vi "UNITEST MAIN v2.0.vi"() -> ()   [LabVIEW 2025] (continued)
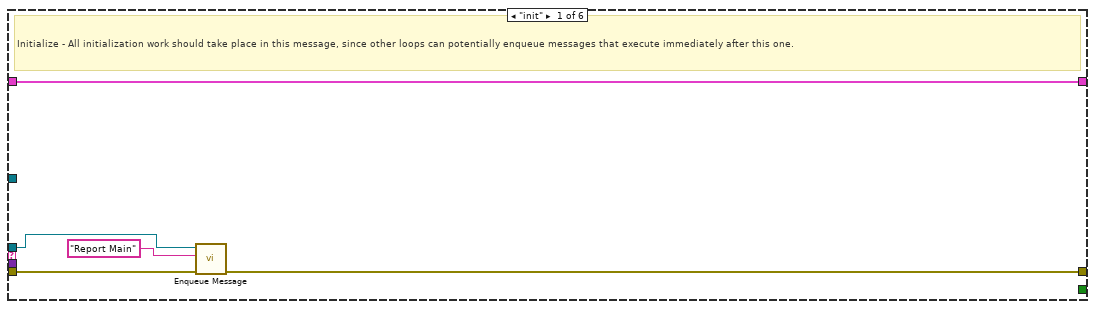
[diagram p2: hidden frame]
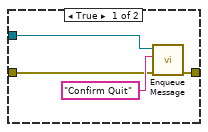
[diagram p3: hidden frame]
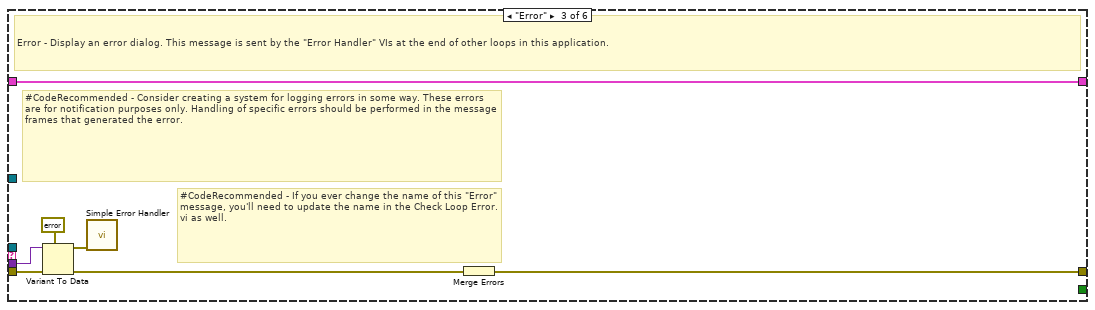
[diagram p4: hidden frame]
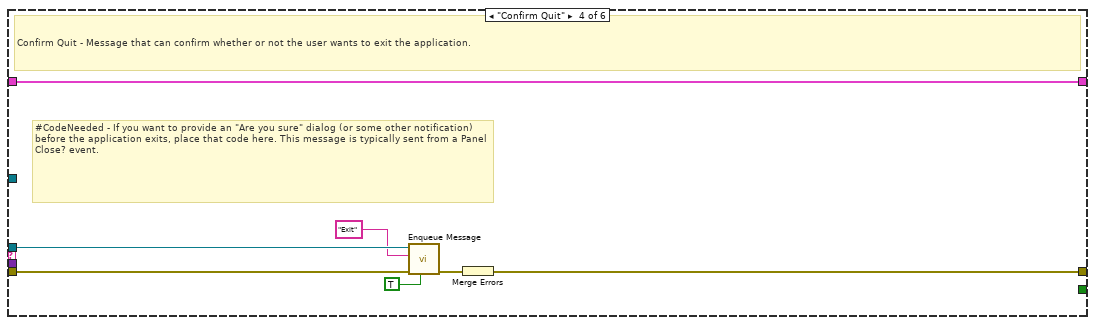
[diagram p5: hidden frame]
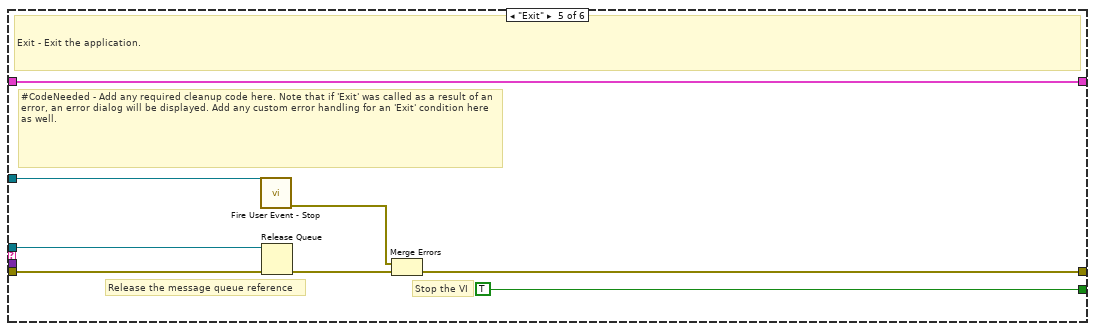
[diagram p6: hidden frame]
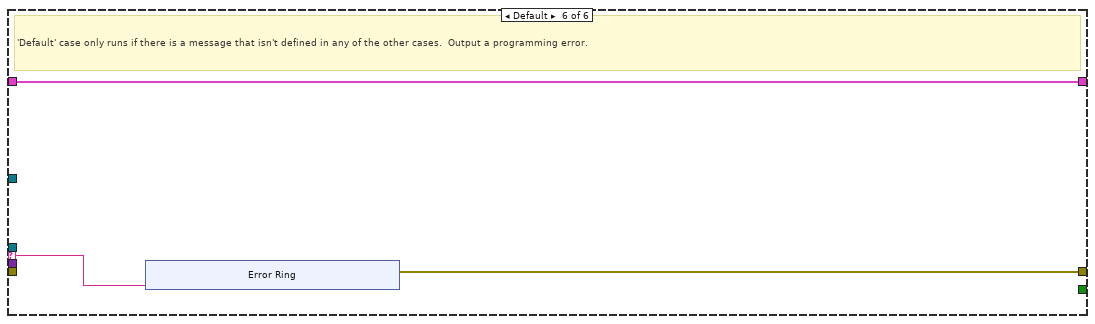
[diagram p7: hidden frame]
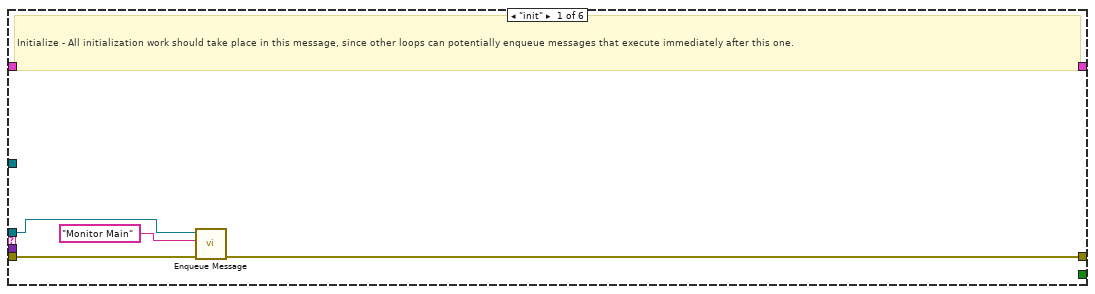
[diagram p8: hidden frame]
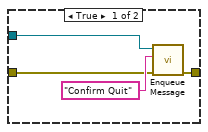
[diagram p9: hidden frame]
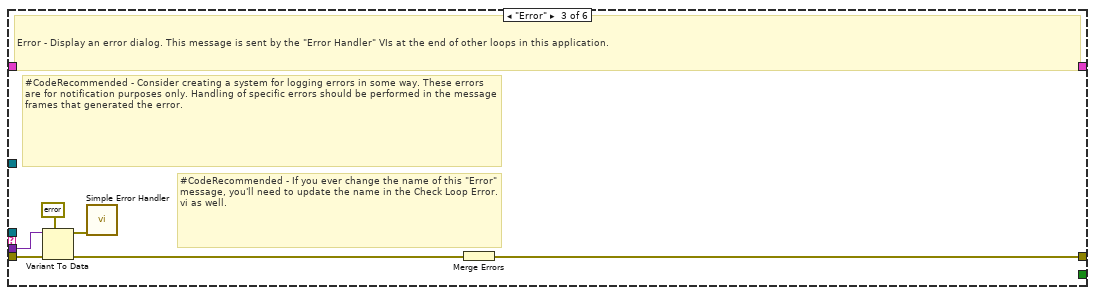
[diagram p10: hidden frame]
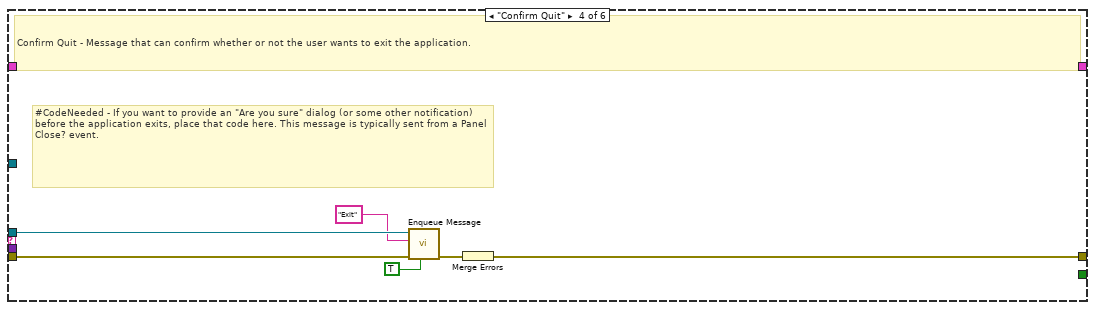
[diagram p11: hidden frame]
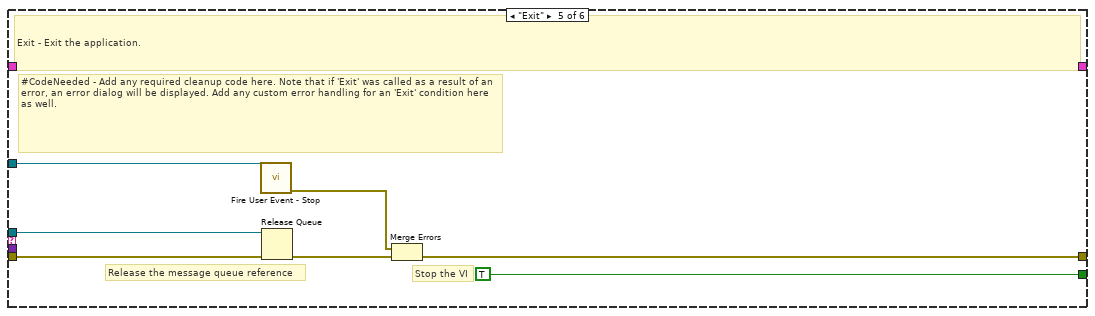
[diagram p12: hidden frame]
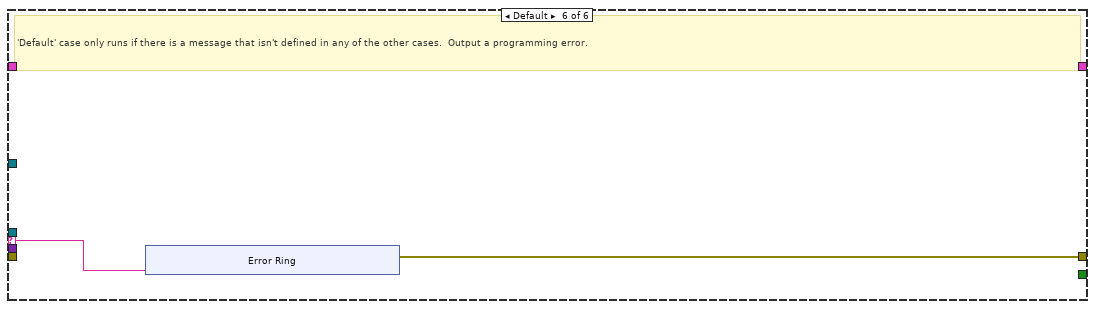
[diagram p13: hidden frame]
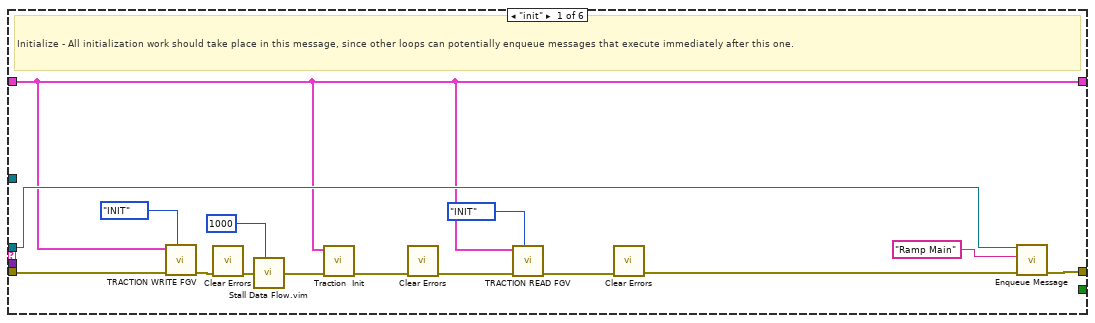
[diagram p14: hidden frame]
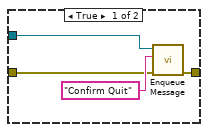
[diagram p16: hidden frame]
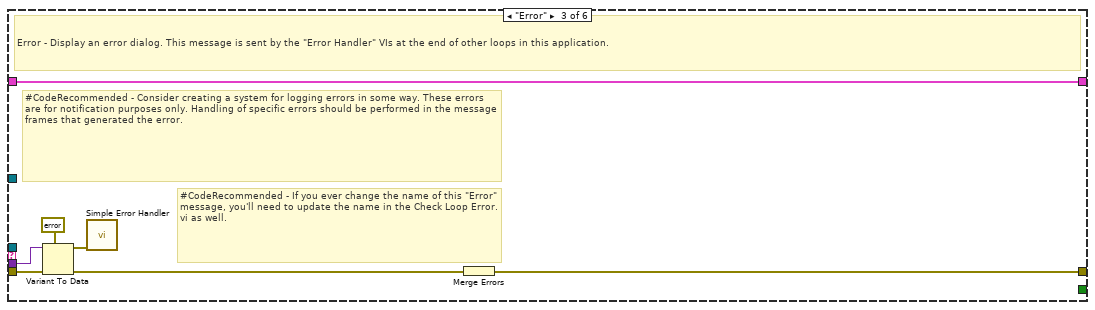
[diagram p17: hidden frame]
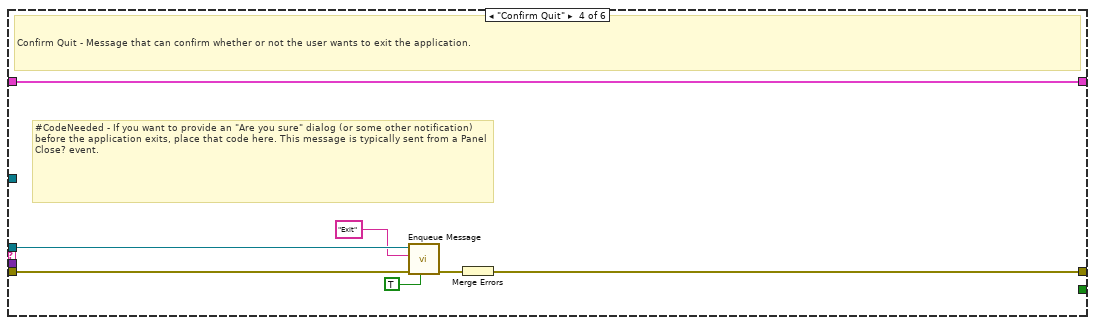
[diagram p18: hidden frame]
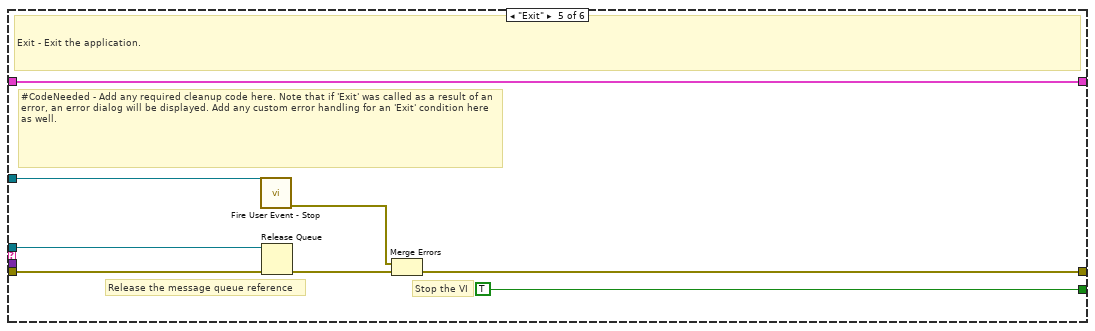
[diagram p19: hidden frame]
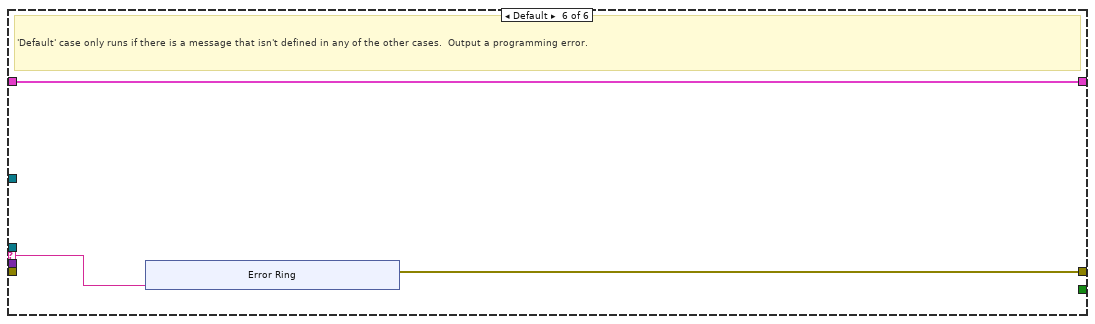
[diagram p20: hidden frame]
        n1992 = call "Traction Receipe Main.vi"("error in (no error)"=w3295, "main ref"=w3292) -> ("error out"=w3294:errorcluster)  [unwired: 9 in]
        n1993 = local write "Traction Receipe Update Details"(FALSE ("Traction Step Update Details")) -> ()
        n1994 = call "DATA ENCRYPT STRING FILE WRITE.vi"("error in (no error)"=w3294, "User Action"="User Pressed  Traction Update Details ", "main ref"=w3292) -> ("error out"=w3293:errorcluster)  [unwired: 6 in, 1 out]
      }
      frame "Acoustic Emission 3" {
        n1995 = Unbundle By Name(w3297) -> ("Environmental control.Acoustic Emission 3"=w3300:refnum<vi>)
        n1996 = property on="Property Node" class="Bool (strict)"(reference=w3300) -> (reference out=w3298:refnum<vi>, error out=w3299:errorcluster, "Value"=w3296:bool)  [unwired: 1 in]
        n1997 = Close Reference(reference=w3298, error in (no error)=w3299) -> ()  [unwired: 1 out]
        n1998 = case shown="True" w3296 {
          tunnel: w3297 -> [w3304 w3309]
          frame True {
            n1999 = Unbundle By Name(w3304) -> ("Acquostic.Gains"=w3306:refnum<vi>)
            n2000 = property class="RadioBtnsControl (strict)"(reference=w3306, "Visible"=TRUE) -> (reference out=w3308:refnum<vi>, error out=w3307:errorcluster)  [unwired: 1 in]
            n2001 = Close Reference(reference=w3308, error in (no error)=w3307) -> ()  [unwired: 1 out]
          }
          frame False {
            n2002 = Unbundle By Name(w3309) -> ("Acquostic.Gains"=w3311:refnum<vi>)
            n2003 = property class="RadioBtnsControl (strict)"(reference=w3311, "Visible"=FALSE) -> (reference out=w3313:refnum<vi>, error out=w3312:errorcluster)  [unwired: 1 in]
            n2004 = Close Reference(reference=w3313, error in (no error)=w3312) -> ()  [unwired: 1 out]
          }
        }
        n2005 = call "DATA ENCRYPT STRING FILE WRITE.vi"("error in (no error)"=w3303, "User Action"="User Pressed  on  Acuostic in Environmental Screen", "main ref"=w3297) -> ("error out"=w3302:errorcluster)  [unwired: 6 in, 1 out]
      }
      frame "Report" {
        n2006 = call "REPORT GENERATION FOR PYTHON.vi"("error in (no error)"=w3319, "main ref"=w3316) -> ("error out"=w3318:errorcluster)  [unwired: 9 in]
        n2007 = local write "Report"(FALSE ("Report")) -> ()
        n2008 = call "DATA ENCRYPT STRING FILE WRITE.vi"("error in (no error)"=w3318, "User Action"="User Pressed Report ", "main ref"=w3316) -> ("error out"=w3317:errorcluster)  [unwired: 6 in, 1 out]
      }
      frame "Error" {
        # "#CodeRecommended - If you ever change the name of this \"Error\" message, you'll need to update the name in the Check Loop Error.vi as well."
        # "#CodeRecommended - Consider creating a system for logging errors in some way. These errors are for notification purposes only. Handling of specific errors should be performed in the message frames that generated the error."
        # "Error - Display an error dialog. This message is sent by the \"Error Handler\" VIs at the end of other loops in this application."
        n2009 = Variant To Data(error in=w3326, type=errorcluster {"status"=FALSE, "code"=0, "source"=""} ("error constant"), Variant=w3324) -> (data=w3322:errorcluster, error out=w3321:errorcluster)
        n2010 = call <vilib>:"Simple Error Handler.vi"("error in (no error)"=w3322) -> ()  [unwired: 4 in, 5 out]
        n2011 = Merge Errors(w3321) -> (w3320:errorcluster)
      }
      frame "Confirm Quit" {
        # "#CodeNeeded - If you want to provide an \"Are you sure\" dialog (or some other notification) before the application exits, place that code here. This message is typically sent from a Panel Close? event."
        # "Confirm Quit - Message that can confirm whether or not the user wants to exit the application."
        n2012 = call-poly "Enqueue Message.vi"("Priority Message? (F)"=TRUE, "error in (no error)"=w3333, "Message"="Exit", "Message Queue"=w3330) -> ("error out"=w3331:errorcluster)  [unwired: 6 in, 1 out]
        n2013 = Merge Errors(w3331) -> (w3332:errorcluster)
      }
      frame "Exit" {
        # "Stop the VI"
        # "Release the message queue reference"
        # "#CodeNeeded - Add any required cleanup code here. Note that if 'Exit' was called as a result of an error, an error dialog will be displayed. Add any custom error handling for an 'Exit' condition here as well."
        # "Exit - Exit the application."
        n2014 = call "Fire User Event - Stop.vi"("User Event - Stop"=w3336) -> ("error out"=w3335:errorcluster)  [unwired: 10 in]
        n2015 = Release Queue(queue=w3341, error in (no error)=w3334) -> (error out=w3338:errorcluster)  [unwired: 1 in, 2 out]
        n2016 = Merge Errors(w3335, w3338) -> (w3337:errorcluster)
      }
      frame Default {
        # "'Default' case only runs if there is a message that isn't defined in any of the other cases.  Output a programming error."
        n2017 = xnode ("Error Ring")("parameter 0"=w3342) -> ("error out"=w3343:errorcluster)
      }
    }
    n2018 = call "LAB-IQ Error Handler - Message Handling Loop.vi"("error in (no error)"=w1944, "Message Queue"=w1946) -> ("dup error in"=w1945:errorcluster)  [unwired: 8 in, 1 out]
  }
  n2019 = timed-loop "Timed Loop" {
    shift-right: [w3362] -> _
    shift-left: w9 -> [w3363]
    tunnel: [w3356] -> w52
    tunnel: w51 -> [w3354]
    tunnel: w6 -> [w3353]
    tunnel: w10 -> [w3352]
    timing: w28 -> [_]
    timing-out: [_] -> w27
    stop <- w3361 stop-if-true
    # "Load  Handling Loop"
    n2020 = node-c288() -> ()  [unwired: 1 in, 1 out]
    n2021 = call "Dequeue Message.vi"("error in (no error)"=w3353, "Message Queue"=w3354) -> ("error out"=w3360:errorcluster, "Message Data"=w3358:variant, "Message"=w3359:string, "dup Message Queue"=w3357:refnum<queue>)  [unwired: 6 in]
    n2022 = case "Message Cases" shown="\"Load Main\"" w3359 {
      selector: w3359 -> [_ _ _ _ _ w3419]
      tunnel: w3357 -> [w3366 w3379 _ w3408 w3418 _]
      tunnel: w3360 -> [w3369 w3377 w3395 w3410 w3412 _]
      tunnel: [w3370 w3380 w3389 w3396 w3414 w3420] -> w3355
      tunnel: w3363 -> [w3368 w3372 w3394 w3405 w3417 w3421]
      tunnel: [w3368 w3372 w3394 w3405 w3417 w3421] -> w3362
      tunnel: [_ _ _ _ TRUE _] -> w3361
      tunnel: w3358 -> [_ _ w3393 _ _ _]
      tunnel: w3352 -> [_ _ _ _ w3411 _]
      frame "init" {
        # "Bundle control references and a sample string value."
        # "Initialize - All initialization work should take place in this message, since other loops can potentially enqueue messages that execute immediately after this one."
        n2023 = call-poly "Enqueue Message.vi"("error in (no error)"=w3369, "Message"="Load Main", "Message Queue"=w3366) -> ("error out"=w3370:errorcluster)  [unwired: 7 in, 1 out]
      }
      frame "Load Main" {
        n2024 = call "LOAD CELL READ.vi"("error in (no error)"=w3377, "main ref"=w3372) -> ("error out"=w3373:errorcluster)  [unwired: 9 in]
        n2025 = call <vilib>:"Clear Errors.vi"("error in (no error)"=w3373) -> ("error out"=w3371:errorcluster)  [unwired: 5 in, 1 out]
        n2026 = Unbundle By Name(w3372) -> ("Main Home Screen.EXIT"=w3378:refnum<vi>)
        n2027 = property on="Property Node" class="Bool (strict)"(reference=w3378) -> (reference out=w3375:refnum<vi>, error out=w3376:errorcluster, "Value"=w3374:bool)  [unwired: 1 in]
        n2028 = Close Reference(reference=w3375, error in (no error)=w3376) -> ()  [unwired: 1 out]
        n2029 = case shown="False" w3374 {
          tunnel: [w3383 w3387] -> w3380
          tunnel: w3379 -> [w3382 w3386]
          tunnel: w3371 -> [w3381 w3385]
          frame True {
            n2030 = call-poly "Enqueue Message.vi"("error in (no error)"=w3381, "Message"="Confirm Quit", "Message Queue"=w3382) -> ("error out"=w3383:errorcluster)  [unwired: 7 in, 1 out]
          }
          frame False {
            n2031 = call-poly "Enqueue Message.vi"("error in (no error)"=w3385, "Message"="Load Main", "Message Queue"=w3386) -> ("error out"=w3387:errorcluster)  [unwired: 7 in, 1 out]
          }
        }
      }
      frame "Error" {
        # "#CodeRecommended - If you ever change the name of this \"Error\" message, you'll need to update the name in the Check Loop Error.vi as well."
        # "#CodeRecommended - Consider creating a system for logging errors in some way. These errors are for notification purposes only. Handling of specific errors should be performed in the message frames that generated the error."
        # "Error - Display an error dialog. This message is sent by the \"Error Handler\" VIs at the end of other loops in this application."
        n2032 = Variant To Data(error in=w3395, type=errorcluster {"status"=FALSE, "code"=0, "source"=""} ("error constant"), Variant=w3393) -> (data=w3391:errorcluster, error out=w3390:errorcluster)
        n2033 = call <vilib>:"Simple Error Handler.vi"("error in (no error)"=w3391) -> ()  [unwired: 4 in, 5 out]
        n2034 = Merge Errors(w3390) -> (w3389:errorcluster)
      }
      frame "Confirm Quit" {
        # "#CodeNeeded - If you want to provide an \"Are you sure\" dialog (or some other notification) before the application exits, place that code here. This message is typically sent from a Panel Close? event."
        # "Confirm Quit - Message that can confirm whether or not the user wants to exit the application."
        n2035 = call-poly "Enqueue Message.vi"("Priority Message? (F)"=TRUE, "error in (no error)"=w3410, "Message"="Exit", "Message Queue"=w3408) -> ("error out"=w3409:errorcluster)  [unwired: 6 in, 1 out]
        n2036 = Merge Errors(w3409) -> (w3401:errorcluster)
        n2037 = call <vilib>:"Clear Errors.vi"("error in (no error)"=w3401) -> ("error out"=w3397:errorcluster)  [unwired: 5 in, 1 out]
        n2038 = call "LOAD CELL FGV MAIN.vi"("Enum"=T32."UNINITIAL", "error in (no error)"=w3397, "main ref"=w3405) -> ("error IO"=w3404:errorcluster)  [unwired: 8 in]
        n2039 = call "Stall Data Flow.vim"("value in"=w3404, "milliseconds to wait"=u32 1000) -> ("value out"=w3399:errorcluster)  [unwired: 1 out]
        n2040 = call "LOAD CELL FGV MAIN.vi"("Enum"=T32."DELETEHANDLE", "error in (no error)"=w3399, "main ref"=w3405) -> ("error IO"=w3400:errorcluster)  [unwired: 8 in]
        n2041 = call <vilib>:"Clear Errors.vi"("error in (no error)"=w3400) -> ("error out"=w3396:errorcluster)  [unwired: 5 in, 1 out]
      }
      frame "Exit" {
        # "Stop the VI"
        # "Release the message queue reference"
        # "#CodeNeeded - Add any required cleanup code here. Note that if 'Exit' was called as a result of an error, an error dialog will be displayed. Add any custom error handling for an 'Exit' condition here as well."
        # "Exit - Exit the application."
        n2042 = call "Fire User Event - Stop.vi"("User Event - Stop"=w3411) -> ("error out"=w3413:errorcluster)  [unwired: 10 in]
        n2043 = Release Queue(queue=w3418, error in (no error)=w3412) -> (error out=w3415:errorcluster)  [unwired: 1 in, 2 out]
        n2044 = Merge Errors(w3413, w3415) -> (w3414:errorcluster)
      }
      frame Default {
        # "'Default' case only runs if there is a message that isn't defined in any of the other cases.  Output a programming error."
        n2045 = xnode ("Error Ring")("parameter 0"=w3419) -> ("error out"=w3420:errorcluster)
      }
    }
    n2046 = call "LAB-IQ Error Handler - Message Handling Loop.vi"("error in (no error)"=w3355, "Message Queue"=w3357) -> ("dup error in"=w3356:errorcluster)  [unwired: 8 in, 1 out]
    n2047 = node-c288() -> ()  [unwired: 1 in, 1 out]
  }
  n2048 = timed-loop "Timed Loop" {
    shift-right: [w3429] -> _
    shift-left: w9 -> [w3440]
    tunnel: [w3434] -> w49
    tunnel: w50 -> [w3432]
    tunnel: w6 -> [w3431]
    tunnel: w10 -> [w3430]
    timing: w30 -> [_]
    timing-out: [_] -> w29
    stop <- w3439 stop-if-true
    # "Sway Motor  Handling Loop"
    n2049 = node-c288() -> ()  [unwired: 1 in, 1 out]
    n2050 = call "Dequeue Message.vi"("error in (no error)"=w3431, "Message Queue"=w3432) -> ("error out"=w3438:errorcluster, "Message Data"=w3436:variant, "Message"=w3437:string, "dup Message Queue"=w3435:refnum<queue>)  [unwired: 6 in]
    n2051 = case "Message Cases" shown="\"Sway Main\"" w3437 {
      selector: w3437 -> [_ _ _ _ _ w3526]
      tunnel: w3435 -> [w3454 w3483 _ w3513 w3525 _]
      tunnel: w3438 -> [w3456 w3466 w3510 w3517 w3519 _]
      tunnel: [w3457 w3484 w3504 w3515 w3521 w3527] -> w3433
      tunnel: w3440 -> [w3444 w3461 w3509 w3516 w3524 w3528]
      tunnel: [w3444 w3461 w3509 w3516 w3524 w3528] -> w3429
      tunnel: [_ _ _ _ TRUE _] -> w3439
      tunnel: w3436 -> [_ _ w3508 _ _ _]
      tunnel: w3430 -> [_ _ _ _ w3518 _]
      frame "init" {
        # "Initialize - All initialization work should take place in this message, since other loops can potentially enqueue messages that execute immediately after this one."
        n2052 = call "SWAY WRITE FGV.vi"("Enum - Menu"=Sway_Write_enum."INIT", "error in (no error)"=w3456, "main ref"=w3444) -> ("error out"=w3453:errorcluster)  [unwired: 8 in]
        n2053 = call <vilib>:"Clear Errors.vi"("error in (no error)"=w3453) -> ("error out"=w3447:errorcluster)  [unwired: 5 in, 1 out]
        n2054 = call "Stall Data Flow.vim"("value in"=w3447, "milliseconds to wait"=u32 1000) -> ("value out"=w3451:errorcluster)  [unwired: 1 out]
        n2055 = call "Sway Init.vi"("error in (no error)"=w3451, "main ref"=w3444) -> ("error out"=w3448:errorcluster)  [unwired: 9 in]
        n2056 = call <vilib>:"Clear Errors.vi"("error in (no error)"=w3448) -> ("error out"=w3446:errorcluster)  [unwired: 5 in, 1 out]
        n2057 = call "SWAY READ FGV.vi"("Enum - Menu"=Sway_Right_enum."INIT", "error in (no error)"=w3446, "main ref"=w3444) -> ("error out"=w3445:errorcluster)  [unwired: 7 in, 1 out]
        n2058 = call <vilib>:"Clear Errors.vi"("error in (no error)"=w3445) -> ("error out"=w3449:errorcluster)  [unwired: 5 in, 1 out]
        n2059 = call-poly "Enqueue Message.vi"("error in (no error)"=w3449, "Message"="Sway Main", "Message Queue"=w3454) -> ("error out"=w3457:errorcluster)  [unwired: 7 in, 1 out]
      }
      frame "Sway Main" {
        n2060 = Unbundle By Name(w3461) -> ("Heave AND Surge.Homed"=w3469:refnum<vi>)
        n2061 = Unbundle By Name(w3461) -> ("SWAY.Read SWAY Temp"=w3478:refnum<vi>)
        n2062 = local read "HEAVE ENABLE"() -> (w3473:bool)
        n2063 = property on="Property Node" class="DigNum (strict)"(reference=w3469) -> (reference out=w3471:refnum<vi>, error out=w3470:errorcluster, "Value"=w3460:u8)  [unwired: 1 in]
        n2064 = property on="Property Node" class="Bool (strict)"(reference=w3478) -> (reference out=w3476:refnum<vi>, error out=w3477:errorcluster, "Value"=w3475:bool)  [unwired: 1 in]
        n2065 = Equal?(x=w3473, y=TRUE) -> (x = y?=w3468:bool)
        n2066 = Close Reference(reference=w3471, error in (no error)=w3470) -> ()  [unwired: 1 out]
        n2067 = Equal?(x=w3460, y=u8 1 ("Value")) -> (x = y?=w3458:bool)
        n2068 = Close Reference(reference=w3476, error in (no error)=w3477) -> ()  [unwired: 1 out]
        n2069 = And(x=w3468, y=w3458) -> (x .and. y?=w3467:bool)
        n2070 = case shown="True" w3475 {
          tunnel: w3466 -> [w3491 w3495]
          tunnel: [w3491 w3494] -> w3463
          tunnel: w3461 -> [_ w3493]
          frame False {
          }
          frame True {
            n2071 = call "SWAY READ FGV.vi"("Enum - Menu"=Sway_Right_enum."READ", "error in (no error)"=w3495, "main ref"=w3493) -> ("error out"=w3494:errorcluster)  [unwired: 7 in, 1 out]
          }
        }
        n2072 = case shown="True" w3467 {
          tunnel: w3461 -> [_ w3490]
          tunnel: w3466 -> [w3485 w3489]
          tunnel: [w3485 w3486] -> w3464
          frame False {
          }
          frame True {
            n2073 = call "SWAY HOME.vi"("error in (no error)"=w3489, "Data Cluster"=w3490) -> ("error out"=w3487:errorcluster)  [unwired: 9 in]
            n2074 = local write "HEAVE ENABLE"(FALSE ("HEAVE ENABLE")) -> ()
            n2075 = call <vilib>:"Clear Errors.vi"("error in (no error)"=w3487) -> ("error out"=w3486:errorcluster)  [unwired: 5 in, 1 out]
          }
        }
        n2076 = call "Sway Reinitize.vi"("error in (no error)"=w3463, "Data Cluster"=w3461) -> ("error out"=w3462:errorcluster)  [unwired: 9 in]
        n2077 = Unbundle By Name(w3461) -> ("Main Home Screen.EXIT"=w3482:refnum<vi>)
        n2078 = property on="Property Node" class="Bool (strict)"(reference=w3482) -> (reference out=w3480:refnum<vi>, error out=w3481:errorcluster, "Value"=w3479:bool)  [unwired: 1 in]
        n2079 = call <vilib>:"Clear Errors.vi"("error in (no error)"=w3462) -> ("error out"=w3474:errorcluster)  [unwired: 5 in, 1 out]
        n2080 = Merge Errors(w3474, w3464) -> (w3465:errorcluster)
        n2081 = Close Reference(reference=w3480, error in (no error)=w3481) -> ()  [unwired: 1 out]
        n2082 = case shown="False" w3479 {
          tunnel: [w3498 w3502] -> w3484
          tunnel: w3483 -> [w3497 w3501]
          tunnel: w3465 -> [w3496 w3500]
          frame True {
            n2083 = call-poly "Enqueue Message.vi"("error in (no error)"=w3496, "Message"="Confirm Quit", "Message Queue"=w3497) -> ("error out"=w3498:errorcluster)  [unwired: 7 in, 1 out]
          }
          frame False {
            n2084 = call-poly "Enqueue Message.vi"("error in (no error)"=w3500, "Message"="Sway Main", "Message Queue"=w3501) -> ("error out"=w3502:errorcluster)  [unwired: 7 in, 1 out]
          }
        }
      }
      frame "Error" {
        # "#CodeRecommended - If you ever change the name of this \"Error\" message, you'll need to update the name in the Check Loop Error.vi as well."
        # "#CodeRecommended - Consider creating a system for logging errors in some way. These errors are for notification purposes only. Handling of specific errors should be performed in the message frames that generated the error."
        # "Error - Display an error dialog. This message is sent by the \"Error Handler\" VIs at the end of other loops in this application."
        n2085 = Variant To Data(error in=w3510, type=errorcluster {"status"=FALSE, "code"=0, "source"=""} ("error constant"), Variant=w3508) -> (data=w3506:errorcluster, error out=w3505:errorcluster)
        n2086 = call <vilib>:"Simple Error Handler.vi"("error in (no error)"=w3506) -> ()  [unwired: 4 in, 5 out]
        n2087 = Merge Errors(w3505) -> (w3504:errorcluster)
      }
      frame "Confirm Quit" {
        # "#CodeNeeded - If you want to provide an \"Are you sure\" dialog (or some other notification) before the application exits, place that code here. This message is typically sent from a Panel Close? event."
        # "Confirm Quit - Message that can confirm whether or not the user wants to exit the application."
        n2088 = call-poly "Enqueue Message.vi"("Priority Message? (F)"=TRUE, "error in (no error)"=w3517, "Message"="Exit", "Message Queue"=w3513) -> ("error out"=w3514:errorcluster)  [unwired: 6 in, 1 out]
        n2089 = Merge Errors(w3514) -> (w3515:errorcluster)
      }
      frame "Exit" {
        # "Stop the VI"
        # "Release the message queue reference"
        # "#CodeNeeded - Add any required cleanup code here. Note that if 'Exit' was called as a result of an error, an error dialog will be displayed. Add any custom error handling for an 'Exit' condition here as well."
        # "Exit - Exit the application."
        n2090 = call "Fire User Event - Stop.vi"("User Event - Stop"=w3518) -> ("error out"=w3520:errorcluster)  [unwired: 10 in]
        n2091 = Release Queue(queue=w3525, error in (no error)=w3519) -> (error out=w3522:errorcluster)  [unwired: 1 in, 2 out]
        n2092 = Merge Errors(w3520, w3522) -> (w3521:errorcluster)
      }
      frame Default {
        # "'Default' case only runs if there is a message that isn't defined in any of the other cases.  Output a programming error."
        n2093 = xnode ("Error Ring")("parameter 0"=w3526) -> ("error out"=w3527:errorcluster)
      }
    }
    n2094 = call "LAB-IQ Error Handler - Message Handling Loop.vi"("error in (no error)"=w3433, "Message Queue"=w3435) -> ("dup error in"=w3434:errorcluster)  [unwired: 8 in, 1 out]
    n2095 = node-c288() -> ()  [unwired: 1 in, 1 out]
  }
  n2096 = timed-loop {
    shift-right: [w3537] -> _
    shift-left: w9 -> [w3556]
    tunnel: [w3550] -> w23
    tunnel: w46 -> [w3548]
    tunnel: w6 -> [w3547]
    tunnel: w10 -> [w3546]
    timing: w2 -> [_]
    timing-out: [_] -> w1
    stop <- w3555 stop-if-true
    # "Ramp Motor  Handling Loop"
    n2097 = node-c288() -> ()  [unwired: 1 in, 1 out]
    n2098 = call "Dequeue Message.vi"("error in (no error)"=w3547, "Message Queue"=w3548) -> ("error out"=w3554:errorcluster, "Message Data"=w3552:variant, "Message"=w3553:string, "dup Message Queue"=w3551:refnum<queue>)  [unwired: 6 in]
    n2099 = case "Message Cases" shown="\"Ramp Main\"" w3553 {
      selector: w3553 -> [_ _ _ _ _ w3628]
      tunnel: w3551 -> [w3572 w3588 _ w3615 w3627 _]
      tunnel: w3554 -> [w3574 w3586 w3612 w3619 w3621 _]
      tunnel: [w3575 w3589 w3606 w3617 w3623 w3629] -> w3549
      tunnel: w3556 -> [w3563 w3577 w3611 w3618 w3626 w3630]
      tunnel: [w3563 w3577 w3611 w3618 w3626 w3630] -> w3537
      tunnel: [_ _ _ _ TRUE _] -> w3555
      tunnel: w3552 -> [_ _ w3610 _ _ _]
      tunnel: w3546 -> [_ _ _ _ w3620 _]
      frame "init" {
        # "Initialize - All initialization work should take place in this message, since other loops can potentially enqueue messages that execute immediately after this one."
        n2100 = call "TRACTION WRITE FGV.vi"("Enum - Menu"=Traction_Write_enum."INIT", "error in (no error)"=w3574, "main ref"=w3563) -> ("error out"=w3571:errorcluster)  [unwired: 8 in]
        n2101 = call <vilib>:"Clear Errors.vi"("error in (no error)"=w3571) -> ("error out"=w3569:errorcluster)  [unwired: 5 in, 1 out]
        n2102 = call "Stall Data Flow.vim"("value in"=w3569, "milliseconds to wait"=u32 1000) -> ("value out"=w3568:errorcluster)  [unwired: 1 out]
        n2103 = call "Traction  Init.vi"("error in (no error)"=w3568, "main ref"=w3563) -> ("error out"=w3566:errorcluster)  [unwired: 9 in]
        n2104 = call <vilib>:"Clear Errors.vi"("error in (no error)"=w3566) -> ("error out"=w3565:errorcluster)  [unwired: 5 in, 1 out]
        n2105 = call "TRACTION READ FGV.vi"("Enum - Menu"=Traction_Read_enum."INIT", "error in (no error)"=w3565, "main ref"=w3563) -> ("error out"=w3564:errorcluster)  [unwired: 7 in, 1 out]
        n2106 = call <vilib>:"Clear Errors.vi"("error in (no error)"=w3564) -> ("error out"=w3562:errorcluster)  [unwired: 5 in, 1 out]
        n2107 = call-poly "Enqueue Message.vi"("error in (no error)"=w3562, "Message"="Ramp Main", "Message Queue"=w3572) -> ("error out"=w3575:errorcluster)  [unwired: 7 in, 1 out]
      }
      frame "Ramp Main" {
        n2108 = Unbundle By Name(w3577) -> ("Traction.Read TRACTION Temp"=w3582:refnum<vi>)
        n2109 = property on="Property Node" class="Bool (strict)"(reference=w3582) -> (reference out=w3580:refnum<vi>, error out=w3581:errorcluster, "Value"=w3578:bool)  [unwired: 1 in]
        n2110 = Close Reference(reference=w3580, error in (no error)=w3581) -> ()  [unwired: 1 out]
        n2111 = case shown="True" w3578 {
          tunnel: w3586 -> [w3590 w3597]
          tunnel: [w3590 w3594] -> w3579
          tunnel: w3577 -> [_ w3595]
          tunnel: w3577 -> [_ w3593]
          frame False {
          }
          frame True {
            n2112 = call "TRACTION READ FGV.vi"("Enum - Menu"=Traction_Read_enum."READ", "error in (no error)"=w3597, "main ref"=w3595) -> ("error out"=w3596:errorcluster, "ERROR TEMP"=w3592:bool)  [unwired: 7 in]
            n2113 = call "Traction Reinitize.vi"("error in (no error)"=w3596, "Checkbox"=w3592, "Data Cluster"=w3593) -> ("error out"=w3594:errorcluster)  [unwired: 8 in]
          }
        }
        n2114 = Unbundle By Name(w3577) -> ("Main Home Screen.EXIT"=w3587:refnum<vi>)
        n2115 = call <vilib>:"Clear Errors.vi"("error in (no error)"=w3579) -> ("error out"=w3576:errorcluster)  [unwired: 5 in, 1 out]
        n2116 = property on="Property Node" class="Bool (strict)"(reference=w3587) -> (reference out=w3584:refnum<vi>, error out=w3585:errorcluster, "Value"=w3583:bool)  [unwired: 1 in]
        n2117 = case shown="False" w3583 {
          tunnel: [w3600 w3604] -> w3589
          tunnel: w3588 -> [w3599 w3603]
          tunnel: w3576 -> [w3598 w3602]
          frame True {
            n2118 = call-poly "Enqueue Message.vi"("error in (no error)"=w3598, "Message"="Confirm Quit", "Message Queue"=w3599) -> ("error out"=w3600:errorcluster)  [unwired: 7 in, 1 out]
          }
          frame False {
            n2119 = call-poly "Enqueue Message.vi"("error in (no error)"=w3602, "Message"="Ramp Main", "Message Queue"=w3603) -> ("error out"=w3604:errorcluster)  [unwired: 7 in, 1 out]
          }
        }
        n2120 = Close Reference(reference=w3584, error in (no error)=w3585) -> ()  [unwired: 1 out]
      }
      frame "Error" {
        # "#CodeRecommended - If you ever change the name of this \"Error\" message, you'll need to update the name in the Check Loop Error.vi as well."
        # "#CodeRecommended - Consider creating a system for logging errors in some way. These errors are for notification purposes only. Handling of specific errors should be performed in the message frames that generated the error."
        # "Error - Display an error dialog. This message is sent by the \"Error Handler\" VIs at the end of other loops in this application."
        n2121 = Variant To Data(error in=w3612, type=errorcluster {"status"=FALSE, "code"=0, "source"=""} ("error constant"), Variant=w3610) -> (data=w3608:errorcluster, error out=w3607:errorcluster)
        n2122 = call <vilib>:"Simple Error Handler.vi"("error in (no error)"=w3608) -> ()  [unwired: 4 in, 5 out]
        n2123 = Merge Errors(w3607) -> (w3606:errorcluster)
      }
      frame "Confirm Quit" {
        # "#CodeNeeded - If you want to provide an \"Are you sure\" dialog (or some other notification) before the application exits, place that code here. This message is typically sent from a Panel Close? event."
        # "Confirm Quit - Message that can confirm whether or not the user wants to exit the application."
        n2124 = call-poly "Enqueue Message.vi"("Priority Message? (F)"=TRUE, "error in (no error)"=w3619, "Message"="Exit", "Message Queue"=w3615) -> ("error out"=w3616:errorcluster)  [unwired: 6 in, 1 out]
        n2125 = Merge Errors(w3616) -> (w3617:errorcluster)
      }
      frame "Exit" {
        # "Stop the VI"
        # "Release the message queue reference"
        # "#CodeNeeded - Add any required cleanup code here. Note that if 'Exit' was called as a result of an error, an error dialog will be displayed. Add any custom error handling for an 'Exit' condition here as well."
        # "Exit - Exit the application."
        n2126 = call "Fire User Event - Stop.vi"("User Event - Stop"=w3620) -> ("error out"=w3622:errorcluster)  [unwired: 10 in]
        n2127 = Release Queue(queue=w3627, error in (no error)=w3621) -> (error out=w3624:errorcluster)  [unwired: 1 in, 2 out]
        n2128 = Merge Errors(w3622, w3624) -> (w3623:errorcluster)
      }
      frame Default {
        # "'Default' case only runs if there is a message that isn't defined in any of the other cases.  Output a programming error."
        n2129 = xnode ("Error Ring")("parameter 0"=w3628) -> ("error out"=w3629:errorcluster)
      }
    }
    n2130 = call "LAB-IQ Error Handler - Message Handling Loop.vi"("error in (no error)"=w3549, "Message Queue"=w3551) -> ("dup error in"=w3550:errorcluster)  [unwired: 8 in, 1 out]
    n2131 = Unbundle By Name(w3537) -> ("Motion Module.Traction"=w3545:refnum<vi>)
    n2132 = property on="Property Node" class="Bool (strict)"(reference=w3545) -> (reference out=w3543:refnum<vi>, error out=w3544:errorcluster, "Value"=w3542:bool)  [unwired: 1 in]
    n2133 = Close Reference(reference=w3543, error in (no error)=w3544) -> ()  [unwired: 1 out]
    n2134 = Equal?(x=w3542, y=TRUE) -> (x = y?=w3540:bool)
    n2135 = Select(t=i64 10 ("Period"), s=w3540, f=i64 1000) -> (s? t:f=w3536:i64)
    n2136 = node-c288(w3536) -> ()  [unwired: 1 in, 1 out]
  }
  n2137 = while {
    shift-right: [w3648] -> _
    shift-left: w9 -> [w3649]
    tunnel: [w3642] -> w15
    tunnel: w43 -> [w3640]
    tunnel: w6 -> [w3639]
    tunnel: w10 -> [w3638]
    stop <- w3647 stop-if-true
    # "Program  Handling Loop"
    n2138 = call "Dequeue Message.vi"("error in (no error)"=w3639, "Message Queue"=w3640) -> ("error out"=w3646:errorcluster, "Message Data"=w3644:variant, "Message"=w3645:string, "dup Message Queue"=w3643:refnum<queue>)  [unwired: 6 in]
    n2139 = case "Message Cases" shown="\"Program Main\"" w3645 {
      selector: w3645 -> [_ _ _ _ _ w3694]
      tunnel: w3643 -> [w3650 w3662 _ w3681 w3693 _]
      tunnel: w3646 -> [w3653 w3656 w3678 w3685 w3687 _]
      tunnel: [w3654 w3663 w3672 w3683 w3689 w3695] -> w3641
      tunnel: w3649 -> [w3652 w3655 w3677 w3684 w3692 w3696]
      tunnel: [w3652 w3655 w3677 w3684 w3692 w3696] -> w3648
      tunnel: [_ _ _ _ TRUE _] -> w3647
      tunnel: w3644 -> [_ _ w3676 _ _ _]
      tunnel: w3638 -> [_ _ _ _ w3686 _]
      frame "init" {
        # "Initialize - All initialization work should take place in this message, since other loops can potentially enqueue messages that execute immediately after this one."
        n2140 = call-poly "Enqueue Message.vi"("error in (no error)"=w3653, "Message"="Program Main", "Message Queue"=w3650) -> ("error out"=w3654:errorcluster)  [unwired: 7 in, 1 out]
      }
      frame "Program Main" {
        n2141 = call "Main Program Loop Vi.vi"("error in (no error)"=w3656, "Data Cluster"=w3655) -> ("error out"=w3657:errorcluster)  [unwired: 9 in]
        n2142 = Unbundle By Name(w3655) -> ("Main Home Screen.EXIT"=w3661:refnum<vi>)
        n2143 = property on="Property Node" class="Bool (strict)"(reference=w3661) -> (reference out=w3659:refnum<vi>, error out=w3660:errorcluster, "Value"=w3658:bool)  [unwired: 1 in]
        n2144 = case shown="False" w3658 {
          tunnel: [w3666 w3670] -> w3663
          tunnel: w3662 -> [w3665 w3669]
          tunnel: w3657 -> [w3664 w3668]
          frame True {
            n2145 = call-poly "Enqueue Message.vi"("error in (no error)"=w3664, "Message"="Confirm Quit", "Message Queue"=w3665) -> ("error out"=w3666:errorcluster)  [unwired: 7 in, 1 out]
          }
          frame False {
            n2146 = call-poly "Enqueue Message.vi"("error in (no error)"=w3668, "Message"="Program Main", "Message Queue"=w3669) -> ("error out"=w3670:errorcluster)  [unwired: 7 in, 1 out]
          }
        }
        n2147 = Close Reference(reference=w3659, error in (no error)=w3660) -> ()  [unwired: 1 out]
      }
      frame "Error" {
        # "#CodeRecommended - If you ever change the name of this \"Error\" message, you'll need to update the name in the Check Loop Error.vi as well."
        # "#CodeRecommended - Consider creating a system for logging errors in some way. These errors are for notification purposes only. Handling of specific errors should be performed in the message frames that generated the error."
        # "Error - Display an error dialog. This message is sent by the \"Error Handler\" VIs at the end of other loops in this application."
        n2148 = Variant To Data(error in=w3678, type=errorcluster {"status"=FALSE, "code"=0, "source"=""} ("error constant"), Variant=w3676) -> (data=w3674:errorcluster, error out=w3673:errorcluster)
        n2149 = call <vilib>:"Simple Error Handler.vi"("error in (no error)"=w3674) -> ()  [unwired: 4 in, 5 out]
        n2150 = Merge Errors(w3673) -> (w3672:errorcluster)
      }
      frame "Confirm Quit" {
        # "#CodeNeeded - If you want to provide an \"Are you sure\" dialog (or some other notification) before the application exits, place that code here. This message is typically sent from a Panel Close? event."
        # "Confirm Quit - Message that can confirm whether or not the user wants to exit the application."
        n2151 = call-poly "Enqueue Message.vi"("Priority Message? (F)"=TRUE, "error in (no error)"=w3685, "Message"="Exit", "Message Queue"=w3681) -> ("error out"=w3682:errorcluster)  [unwired: 6 in, 1 out]
        n2152 = Merge Errors(w3682) -> (w3683:errorcluster)
      }
      frame "Exit" {
        # "Stop the VI"
        # "Release the message queue reference"
        # "#CodeNeeded - Add any required cleanup code here. Note that if 'Exit' was called as a result of an error, an error dialog will be displayed. Add any custom error handling for an 'Exit' condition here as well."
        # "Exit - Exit the application."
        n2153 = call "Fire User Event - Stop.vi"("User Event - Stop"=w3686) -> ("error out"=w3688:errorcluster)  [unwired: 10 in]
        n2154 = Release Queue(queue=w3693, error in (no error)=w3687) -> (error out=w3690:errorcluster)  [unwired: 1 in, 2 out]
        n2155 = Merge Errors(w3688, w3690) -> (w3689:errorcluster)
      }
      frame Default {
        # "'Default' case only runs if there is a message that isn't defined in any of the other cases.  Output a programming error."
        n2156 = xnode ("Error Ring")("parameter 0"=w3694) -> ("error out"=w3695:errorcluster)
      }
    }
    n2157 = call "LAB-IQ Error Handler - Message Handling Loop.vi"("error in (no error)"=w3641, "Message Queue"=w3643) -> ("dup error in"=w3642:errorcluster)  [unwired: 8 in, 1 out]
  }
  n2158 = while "Timed Loop" {
    shift-right: [w3710] -> _
    shift-left: w9 -> [w3724]
    tunnel: [w3718] -> w14
    tunnel: w42 -> [w3716]
    tunnel: w6 -> [w3715]
    tunnel: w10 -> [w3714]
    stop <- w3723 stop-if-true
    # "Monitor  Handling Loop"
    n2159 = call "Dequeue Message.vi"("error in (no error)"=w3715, "Message Queue"=w3716) -> ("error out"=w3722:errorcluster, "Message Data"=w3720:variant, "Message"=w3721:string, "dup Message Queue"=w3719:refnum<queue>)  [unwired: 6 in]
    n2160 = case "Message Cases" shown="\"Monitor Main\"" w3721 {
      selector: w3721 -> [_ _ _ _ _ w3772]
      tunnel: w3719 -> [w3725 w3740 _ w3759 w3771 _]
      tunnel: w3722 -> [w3728 w3730 w3756 w3763 w3765 _]
      tunnel: [w3729 w3741 w3750 w3761 w3767 w3773] -> w3717
      tunnel: w3724 -> [w3727 w3731 w3755 w3762 w3770 w3774]
      tunnel: [w3727 w3731 w3755 w3762 w3770 w3774] -> w3710
      tunnel: [_ _ _ _ TRUE _] -> w3723
      tunnel: w3720 -> [_ _ w3754 _ _ _]
      tunnel: w3714 -> [_ _ _ _ w3764 _]
      frame "init" {
        # "Initialize - All initialization work should take place in this message, since other loops can potentially enqueue messages that execute immediately after this one."
        n2161 = call-poly "Enqueue Message.vi"("error in (no error)"=w3728, "Message"="Monitor Main", "Message Queue"=w3725) -> ("error out"=w3729:errorcluster)  [unwired: 7 in, 1 out]
      }
      frame "Monitor Main" {
        n2162 = call "Main Monitor Loop.vi"("error in (no error)"=w3730, "main ref"=w3731) -> ("error out"=w3735:errorcluster)  [unwired: 9 in]
        n2163 = call "LOAD SELECTION MAIN CODE.vi"("error in (no error)"=w3730, "main ref"=w3731) -> ("error out"=w3733:errorcluster)  [unwired: 9 in]
        n2164 = call "Trip Log and Trip Monitor.vi"("error in (no error)"=w3730, "main ref"=w3731) -> ("error out"=w3732:errorcluster)  [unwired: 9 in]
        n2165 = Merge Errors(w3735, w3733, w3732) -> (w3734:errorcluster)
        n2166 = Unbundle By Name(w3731) -> ("Main Home Screen.EXIT"=w3739:refnum<vi>)
        n2167 = property on="Property Node" class="Bool (strict)"(reference=w3739) -> (reference out=w3737:refnum<vi>, error out=w3738:errorcluster, "Value"=w3736:bool)  [unwired: 1 in]
        n2168 = case shown="False" w3736 {
          tunnel: [w3744 w3748] -> w3741
          tunnel: w3740 -> [w3743 w3747]
          tunnel: w3734 -> [w3742 w3746]
          frame True {
            n2169 = call-poly "Enqueue Message.vi"("error in (no error)"=w3742, "Message"="Confirm Quit", "Message Queue"=w3743) -> ("error out"=w3744:errorcluster)  [unwired: 7 in, 1 out]
          }
          frame False {
            n2170 = call-poly "Enqueue Message.vi"("error in (no error)"=w3746, "Message"="Monitor Main", "Message Queue"=w3747) -> ("error out"=w3748:errorcluster)  [unwired: 7 in, 1 out]
          }
        }
        n2171 = Close Reference(reference=w3737, error in (no error)=w3738) -> ()  [unwired: 1 out]
      }
      frame "Error" {
        # "#CodeRecommended - If you ever change the name of this \"Error\" message, you'll need to update the name in the Check Loop Error.vi as well."
        # "#CodeRecommended - Consider creating a system for logging errors in some way. These errors are for notification purposes only. Handling of specific errors should be performed in the message frames that generated the error."
        # "Error - Display an error dialog. This message is sent by the \"Error Handler\" VIs at the end of other loops in this application."
        n2172 = Variant To Data(error in=w3756, type=errorcluster {"status"=FALSE, "code"=0, "source"=""} ("error constant"), Variant=w3754) -> (data=w3752:errorcluster, error out=w3751:errorcluster)
        n2173 = call <vilib>:"Simple Error Handler.vi"("error in (no error)"=w3752) -> ()  [unwired: 4 in, 5 out]
        n2174 = Merge Errors(w3751) -> (w3750:errorcluster)
      }
      frame "Confirm Quit" {
        # "#CodeNeeded - If you want to provide an \"Are you sure\" dialog (or some other notification) before the application exits, place that code here. This message is typically sent from a Panel Close? event."
        # "Confirm Quit - Message that can confirm whether or not the user wants to exit the application."
        n2175 = call-poly "Enqueue Message.vi"("Priority Message? (F)"=TRUE, "error in (no error)"=w3763, "Message"="Exit", "Message Queue"=w3759) -> ("error out"=w3760:errorcluster)  [unwired: 6 in, 1 out]
        n2176 = Merge Errors(w3760) -> (w3761:errorcluster)
      }
      frame "Exit" {
        # "Stop the VI"
        # "Release the message queue reference"
        # "#CodeNeeded - Add any required cleanup code here. Note that if 'Exit' was called as a result of an error, an error dialog will be displayed. Add any custom error handling for an 'Exit' condition here as well."
        # "Exit - Exit the application."
        n2177 = call "Fire User Event - Stop.vi"("User Event - Stop"=w3764) -> ("error out"=w3766:errorcluster)  [unwired: 10 in]
        n2178 = Release Queue(queue=w3771, error in (no error)=w3765) -> (error out=w3768:errorcluster)  [unwired: 1 in, 2 out]
        n2179 = Merge Errors(w3766, w3768) -> (w3767:errorcluster)
      }
      frame Default {
        # "'Default' case only runs if there is a message that isn't defined in any of the other cases.  Output a programming error."
        n2180 = xnode ("Error Ring")("parameter 0"=w3772) -> ("error out"=w3773:errorcluster)
      }
    }
    n2181 = Unbundle By Name(w3710) -> ("Environmental control.Acoustic Emission 3"=w3713:refnum<vi>)
    n2182 = property on="Property Node" class="Bool (strict)"(reference=w3713) -> (reference out=w3711:refnum<vi>, error out=w3712:errorcluster, "Value"=w3709:bool)  [unwired: 1 in]
    n2183 = call "LAB-IQ Error Handler - Message Handling Loop.vi"("error in (no error)"=w3717, "Message Queue"=w3719) -> ("dup error in"=w3718:errorcluster)  [unwired: 8 in, 1 out]
    n2184 = Close Reference(reference=w3711, error in (no error)=w3712) -> ()  [unwired: 1 out]
    n2185 = Equal?(x=w3709, y=TRUE) -> (x = y?=w3707:bool)
    n2186 = Select(t=i64 10 ("Period"), s=w3707, f=i64 100) -> (s? t:f=w3704:i64)
    n2187 = Wait Until Next ms Multiple(millisecond multiple=w3704) -> ()  [unwired: 1 out]
  }
  n2188 = Unregister For Events(event registration refnum=w75, error in=w73) -> (error out=w76:errorcluster)
  n2189 = node-c288(w27) -> ()  [unwired: 1 out]
  n2190 = node-c288(w19) -> ()  [unwired: 1 out]
  n2191 = node-c288(w25) -> ()  [unwired: 1 out]
  n2192 = node-c288(w29) -> ()  [unwired: 1 out]
  n2193 = node-c288(w1) -> ()  [unwired: 1 out]
  n2194 = node-c288(w3) -> ()  [unwired: 1 out]
  n2195 = Merge Errors(w76, w79, w52, w49, w47, w32, w23, w17, w16, w15, w14, w12, w13, w5) -> (w77:errorcluster)
  n2196 = call "Destroy User Event - Stop.vi"("error in (no error)"=w77, "User Event - Stop"=w10) -> ("error out"=w74:errorcluster)  [unwired: 9 in]
  n2197 = disable-structure "Conditional Disable Structure" shown="RUN_TIME_ENGINE==True" {
    disable-tunnel: w74 -> [_ _]
    frame condition #0 (active) {
    }
    frame condition #1 {
      # "Call Quit LabVIEW if running as a built application."
      n2198 = Quit LabVIEW() -> ()  [unwired: 1 in]
    }
  }
